vi "TDMS Configure.vi"(8 "error in (no error)":errorcluster, 10 "Max File Size (GB)":dbl, 11 "TDMS File Path":path) -> (0 "error out":errorcluster, 3 "Refnum out":refnum<k34>)   [LabVIEW 2023]
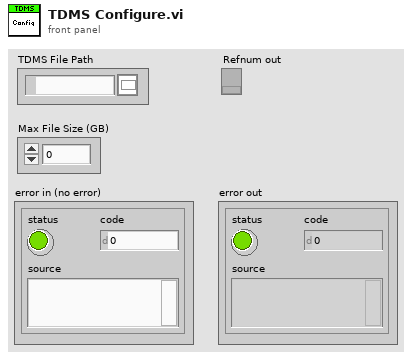
[diagram p1: front panel]
types:
  T1 = enum16{"open", "open or create", "create or replace", "create", "open (read-only)"}
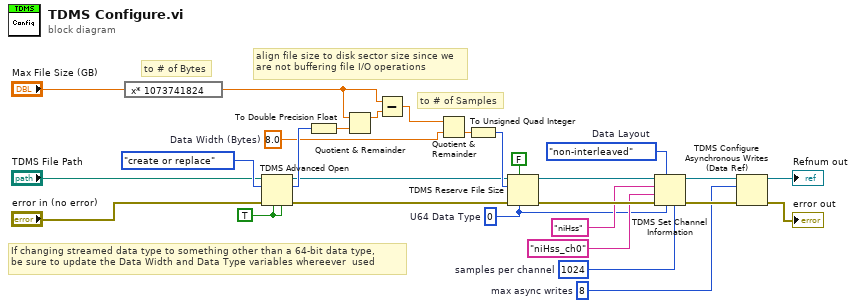
[diagram p0: block diagram]
diagram:
  w9 = TRUE ("disable buffering? (T)")
  w14 = u32 1024  # samples per channel
  w15 = enum16{"non-interleaved", "interleaved"}."non-interleaved"  # Data Layout
  w11 = 8.0  # Data Width (Bytes)
  w6 = u64 0  # U64 Data Type
  w1 = u32 8  # max async writes
  # "If changing streamed data type to something other than a 64-bit data type,\nbe sure to update the Data Width and Data Type variables whereever  used"
  # "align file size to disk sector size since we\nare not buffering file I/O operations"
  # "to # of Samples"
  # "to # of Bytes"
  n1 = expression code="x* 1073741824"("Max File Size (GB)") -> (w19:dbl)
  n2 = TDMS Advanced Open(4:w9, 6:w9, 8:"error in (no error)", 10:T1."create or replace" ("operation (0:open)"), 11:"TDMS File Path") -> (0:w8:errorcluster, 2:w28:u32, 3:w7:refnum<k34>)
  n3 = To Double Precision Float(number=w28) -> (double precision float=w21:dbl)
  n4 = Quotient & Remainder(x=w19, y=w21) -> (x-y*floor(x/y)=w20:dbl)  [unwired: 1 out]
  n5 = Subtract(x=w19, y=w20) -> (x-y=w18:dbl)
  n6 = Quotient & Remainder(x=w18, y=w11) -> (floor(x/y)=w17:dbl)  [unwired: 1 out]
  n7 = To Unsigned Quad Integer(1:w17) -> (0:w10:u64)
  n8 = TDMS Reserve File Size(6:w6, 7:FALSE ("append? (T)"), 8:w8, 10:w10, 11:w7) -> (0:w25:errorcluster, 3:w26:refnum<k34>)
  n9 = TDMS Set Channel Information(4:w14, 6:w6, 7:w15, 8:w25, 9:"niHss_ch0" ("group name (Untitled)"), 10:"niHss" ("group name (Untitled)"), 11:w26) -> (0:w2:errorcluster, 3:w5:refnum<k34>)
  n10 = TDMS Configure Asynchronous Writes (Data Ref)(8:w2, 10:w1, 11:w5) -> (0:→"error out":errorcluster, 3:→"Refnum out":refnum<k34>)  [unwired: 1 in]
